vi "ADC INL_new - Copy.vi"(8 "error in (no error)":errorcluster, 9 "Sequence parameters":string[][](array[string])=[["Min limit", "Max limit", "Register sheet file", "Register Sheet"], ["", "", "CC2600.xls", "TX_BLE;Trim"], ["Reg write (addr;value)", "Operating frequency [Hz]", "", ""], ["NA", "2.44G", "", ""]], 10 "Run type":i32, 11 "Method parameters":T3={"Dev"={"Do not disturb DUT"=FALSE, "XOSC"=32000000.0, "Board type"="", "EM"="", "Configure tempboard"=TRUE, "Device specific info"=[], "Generic Object"=refnum}, "Method"={"Run type"=1, "Test name"="Current LPM2 4", "Comment"="", "Results folder"="", "AFC"=enum."Off", "Method name"="Current LPM2 4", "Method results"={"Excel brief report"=FALSE, "Spotfire report"=FALSE, "Starfish report"=FALSE}, "Operator"="", "Reference time"=timestamp(0 s since 1904-01-01), "AFC delay"=0.0, "Initialization"=enum."Enabled", "MD5 Sum"="", "HW addon board"=enum."None", "AFC Regsheet"="", "AFC Regfile"=path "", "dummy"=0.0}, "Inst"={"Instr"={"PS1"={"Name"="", "GPIB address"="", "VISA session"=""}, "PS2"={"Name"="", "GPIB address"="", "VISA session"=""}, "TC1"={"Name"="", "GPIB address"="", "VISA session"=""}, "TC2"={"Name"="", "GPIB address"="", "VISA session"=""}, "SA1"={"Name"="", "GPIB address"="", "VISA session"=""}, "SA2"={"Name"="", "GPIB address"="", "VISA session"=""}, "SG1"={"Name"="", "GPIB address"="", "VISA session"=""}, "SG2"={"Name"="", "GPIB address"="", "VISA session"=""}, "SG3"={"Name"="", "GPIB address"="", "VISA session"=""}, "MI1"={"Name"="", "GPIB address"="", "VISA session"=""}, "MI2"={"Name"="", "GPIB address"="", "VISA session"=""}, "SW SA"={"Name"="", "Controller addr"=""}, "SW SG"={"Name"="", "Controller addr"=""}, "MI3"={"Name"="", "GPIB address"="", "VISA session"=""}}, "Switchbox"={"RF Path"=0, "Cal compensation"=enum."TX", "Switchbox gain mode"="", "State"=enum."TX"}, "Instr to control (i.e. SA1)"="Default", "Intrument info string"=""}, "Sequence parameters"=[["Weight", "Min Limit", "Max Limit", "Register Sheet", "", "", "", "", "", "", "", "", ""], ["Vital", "", "1", "LPM2", "", "", "", "", "", "", "", "", ""], ["Resolution", "Reg write (addr;value)", "Chip mode", "Range", "", "", "", "", "", "", "", "", ""], ["u", "NA", "", "auto", "", "", "", "", "", "", "", "", ""]], "Cond"={"Temp logged"=25.0, "VDD1_PS1_6V"=-999.0, "VDD2_PS1_25V"=-999.0, "VDD4_PS2_25V"=-999.0, "VDD3_PS2_6V"=-999.0}, "Meas config"={"X-axis inner loop index"=32000000, "Y-axis outer loop index"=32000000, "X-axis"=[], "Y-axis"=[], "X-axis array req size"=32000000, "Y-axis array req size"=32000000, "Param description"=[], "Use meas clust for reporting"=FALSE, "Parameter index (page)"=0, "X-axis name"="", "Y-axis name"=""}} {"Cond"."VDD3_PS2_6V" format="%.3f"; "Cond"."VDD4_PS2_25V" format="%.3f"; "Cond"."VDD2_PS1_25V" format="%.3f"; "Cond"."VDD1_PS1_6V" format="%.3f"; "Method"."dummy" format="%.1p"; "Method"."AFC delay" format="%.1p"; "Dev"."XOSC" format="%.3p"}) -> (0 "error out":errorcluster, 1 "End method error":T2, 2 "Short Results":string[](array[string])=["0.00", "0.00", "0.00", "0.00"], 3 "Result summary":string[][](array[string])=[["Critical", "Output Power@2405 MHz", "-3", "4", "dBm"], ["Critical", "Output Power@2410 MHz", "-3", "4", "dBm"]])   [LabVIEW 2019]
doc: "[AutoDocStart]Performs crystal accuracy measurements. Measures the offset from ideal frequency. Primarily used for tuning XOSC capacitors and verifying XOSC trims.\n\nSweeping parameters: operating frequency, OSC override value and VDDR level\n\nResults: Offset frequency in ppm[AutoDocEnd]"
uses:
  User Lib/Utilities/Cluster definitions/Method input.ctl
  User Lib/Utilities/Cluster definitions/Device specific info.ctl
  User Lib/Utilities/Controls/Automatic Frequency Compensation types.ctl
  User Lib/Utilities/Controls/Method Reports.ctl
  User Lib/Utilities/Cluster definitions/Method Initialization.ctl
  User Lib/Utilities/Controls/HW addon boards.ctl
  User Lib/Utilities/Cluster definitions/Instr clust.ctl
  User Lib/Utilities/Switchbox control/SwitchBox_State._ENUMctl.ctl
  User Lib/Utilities/Cluster definitions/End method error cluster.ctl
  User Lib/Utilities/Cluster definitions/DUT vdd control.ctl
  User Lib/Utilities/Cluster definitions/DUT VDD4.ctl
  User Lib/Utilities/Cluster definitions/DUT VDD3.ctl
  User Lib/Utilities/Cluster definitions/DUT VDD2.ctl
  User Lib/Utilities/Cluster definitions/DUT VDD1.ctl
  User Lib/Generic chip methods/Classes/Generic_EM/Chameleon/Loki/Loki.lvclass
  <vilib>/Utility/error.llb/Clear Errors.vi
  User Lib/Generic chip methods/Classes/Generic_EM/Chameleon/65nm.lvclass
  C:/Kharon/User Lib/Generic chip methods/Classes/Generic_EM/Generic_EM/Generic_EM.lvclass
  User Lib/Generic chip methods/board_to_chip_type.vi
  User Lib/Generic chip methods/Classes/Get_Class_init.vi
  User Lib/Generic chip methods/Classes/Generic_EM/Generic_EM/Generic_EM.lvclass
panel:
  in  "Tab Control":T1(tab)
  out "output cluster":T11={"Average Hits \nper Code "=198.76479217603912, "Min DNL"=-0.30764433555407467, "Min INL"=-0.5231398172109945, "Max INL"=0.7801825995135989, "Max DNL"=0.8022935268616486, "DNL Range"=0.5549689312078616, "INL Range"=0.6516612083622967}
  out "ADC samples":u32[](array[numeric])
  out "Output Response [All DUTs]":u32[][](array[numeric])
  # "°C"
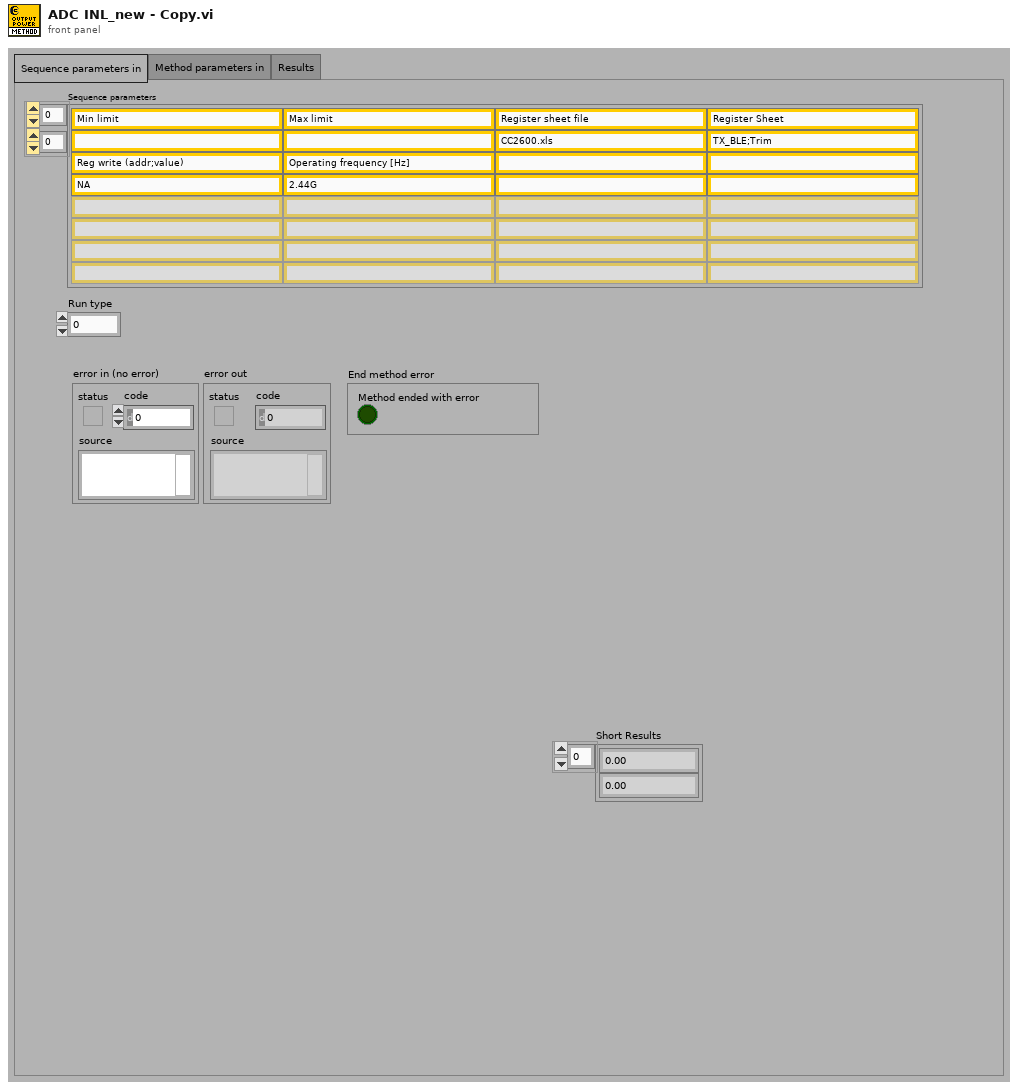
[diagram p1: front panel]
types:
  T1 = enum32{"Sequence parameters in", "Method parameters in", "Results"}
  T2 = typedef "End method error cluster.ctl" = cluster{"Method ended with error":bool}
  T3 = typedef "Method input.ctl" = cluster{"Dev":cluster{"Do not disturb DUT":bool, "XOSC":dbl, "Board type":string, "EM":string, "Configure tempboard":bool, "Device specific info":T4[], "Generic Object":refnum<class>}, "Method":cluster{"Run type":i32, "Test name":string, "Comment":string, "Results folder":string, "AFC":T5, "Method name":string, "Method results":T6, "Operator":string, "Reference time":timestamp, "AFC delay":dbl, "Initialization":T7, "MD5 Sum":string, "HW addon board":T8, "AFC Regsheet":string, "AFC Regfile":path, "dummy":dbl}, "Inst":T9, "Sequence parameters":string[][], "Cond":cluster{"Temp logged":dbl, "VDD1_PS1_6V":dbl, "VDD2_PS1_25V":dbl, "VDD4_PS2_25V":dbl, "VDD3_PS2_6V":dbl}, "Meas config":cluster{"X-axis inner loop index":i32, "Y-axis outer loop index":i32, "X-axis":string[], "Y-axis":string[], "X-axis array req size":i32, "Y-axis array req size":i32, "Param description":string[][], "Use meas clust for reporting":bool, "Parameter index (page)":i32, "X-axis name":string, "Y-axis name":string}}
  T4 = typedef "Device specific info.ctl" = cluster{"EM number":u8, "IP address":string, "Enabled":bool, "Slot no":u8, "RF path":u8, "EM name":string, "Wafer info":string, "AFC frequency ppm":dbl, "Register writes":string[][], "Meas data":string[][][], "Device comment":string}
  T5 = typedef "Automatic Frequency Compensation types.ctl" = enum16{"Off", "Compensate Instrument frequency", "Compensate DUT frequency", "Predictive - Compensate Instrument frequency", "Predictive - Compensate DUT frequency", "Do not skip re-init - Compensate Instrument frequency", "Do not skip re-init - Compensate DUT frequency"}
  T6 = typedef "Method Reports.ctl" = cluster{"Excel brief report":bool, "Spotfire report":bool, "Starfish report":bool}
  T7 = typedef "Method Initialization.ctl" = enum16{"Enabled", "Skip Instr and Device Init", "Enabled with Separate Flash", "Set PS, Device Init and Skip Instr Init", "Skip Device Init"}
  T8 = typedef "HW addon boards.ctl" = enum16{"None", "Current meas 5EM", "Stresstest 10EM"}
  T9 = typedef "Instr clust.ctl" = cluster{"Instr":cluster{"PS1":cluster{"Name":string, "GPIB address":string, "VISA session":refnum<visa-resource-name>}, "PS2":cluster{"Name":string, "GPIB address":string, "VISA session":refnum<visa-resource-name>}, "TC1":cluster{"Name":string, "GPIB address":string, "VISA session":refnum<visa-resource-name>}, "TC2":cluster{"Name":string, "GPIB address":string, "VISA session":refnum<visa-resource-name>}, "SA1":cluster{"Name":string, "GPIB address":string, "VISA session":refnum<visa-resource-name>}, "SA2":cluster{"Name":string, "GPIB address":string, "VISA session":refnum<visa-resource-name>}, "SG1":cluster{"Name":string, "GPIB address":string, "VISA session":refnum<visa-resource-name>}, "SG2":cluster{"Name":string, "GPIB address":string, "VISA session":refnum<visa-resource-name>}, "SG3":cluster{"Name":string, "GPIB address":string, "VISA session":refnum<visa-resource-name>}, "MI1":cluster{"Name":string, "GPIB address":string, "VISA session":refnum<visa-resource-name>}, "MI2":cluster{"Name":string, "GPIB address":string, "VISA session":refnum<visa-resource-name>}, "SW SA":cluster{"Name":string, "Controller addr":string}, "SW SG":cluster{"Name":string, "Controller addr":string}, "MI3":cluster{"Name":string, "GPIB address":string, "VISA session":refnum<visa-resource-name>}}, "Switchbox":cluster{"RF Path":i32, "Cal compensation":enum16{"TX", "RX", "Interferer", "No compensation", "Interferer2"}, "Switchbox gain mode":string, "State":T10}, "Instr to control (i.e. SA1)":string, "Intrument info string":string}
  T10 = typedef "SwitchBox_State._ENUMctl.ctl" = enum16{"TX", "RX", "SP:TX", "SP:RX", "SW:TX", "SW:RX"}
  T11 = cluster{"Average Hits \nper Code ":dbl, "Min DNL":dbl, "Min INL":dbl, "Max INL":dbl, "Max DNL":dbl, "DNL Range":dbl, "INL Range":dbl}
  T12 = cluster{"Path to Save plot":path, "Path to Raw Data plot":path}
  T13 = cluster{"Save INL/DNL Plot(Ramp)":bool, "Save SNR Plot":bool, "Save INL/DNL Plot(Sine)":bool, "Save INL/DNL Raw Data(Ramp)":bool, "Save SNR Raw Data":bool, "Save INL/DNL Raw Data(Sine)":bool, "Save DC Raw data":bool, "Save  Raw Data(Sine)":bool}
  T14 = typedef "DUT vdd control.ctl" = cluster{"VDD4 config":T15, "VDD3 config":T16, "VDD2 config":T17, "VDD1 config":T18}
  T15 = typedef "DUT VDD4.ctl" = u16
  T16 = typedef "DUT VDD3.ctl" = u16
  T17 = typedef "DUT VDD2.ctl" = u16
  T18 = typedef "DUT VDD1.ctl" = u16
  T19 = enum32{"NI Card Settings", "Memory Read Setting", "DC Capture", "ADC Ramp", "ADC Sine", "SNR", "Cap Calibration"}
  T20 = enum32{"Read from Memory", "Read .dat file", "NI Card Capture", "None"}
  T21 = typedef "TFW ResponseData.ctl" = cluster{"errorCode":u32, "executionTime":u32, "processedCmdWord":u32, "responsePar":u32[], "actionCode":u32, "cmdStatus":u16}
  T22 = cluster{"Min INL":dbl, "Max INL":dbl, "Min DNL":dbl, "Max DNL":dbl, "INL Range":dbl, "DNL Range":dbl, "Avg Hits/Code":dbl}
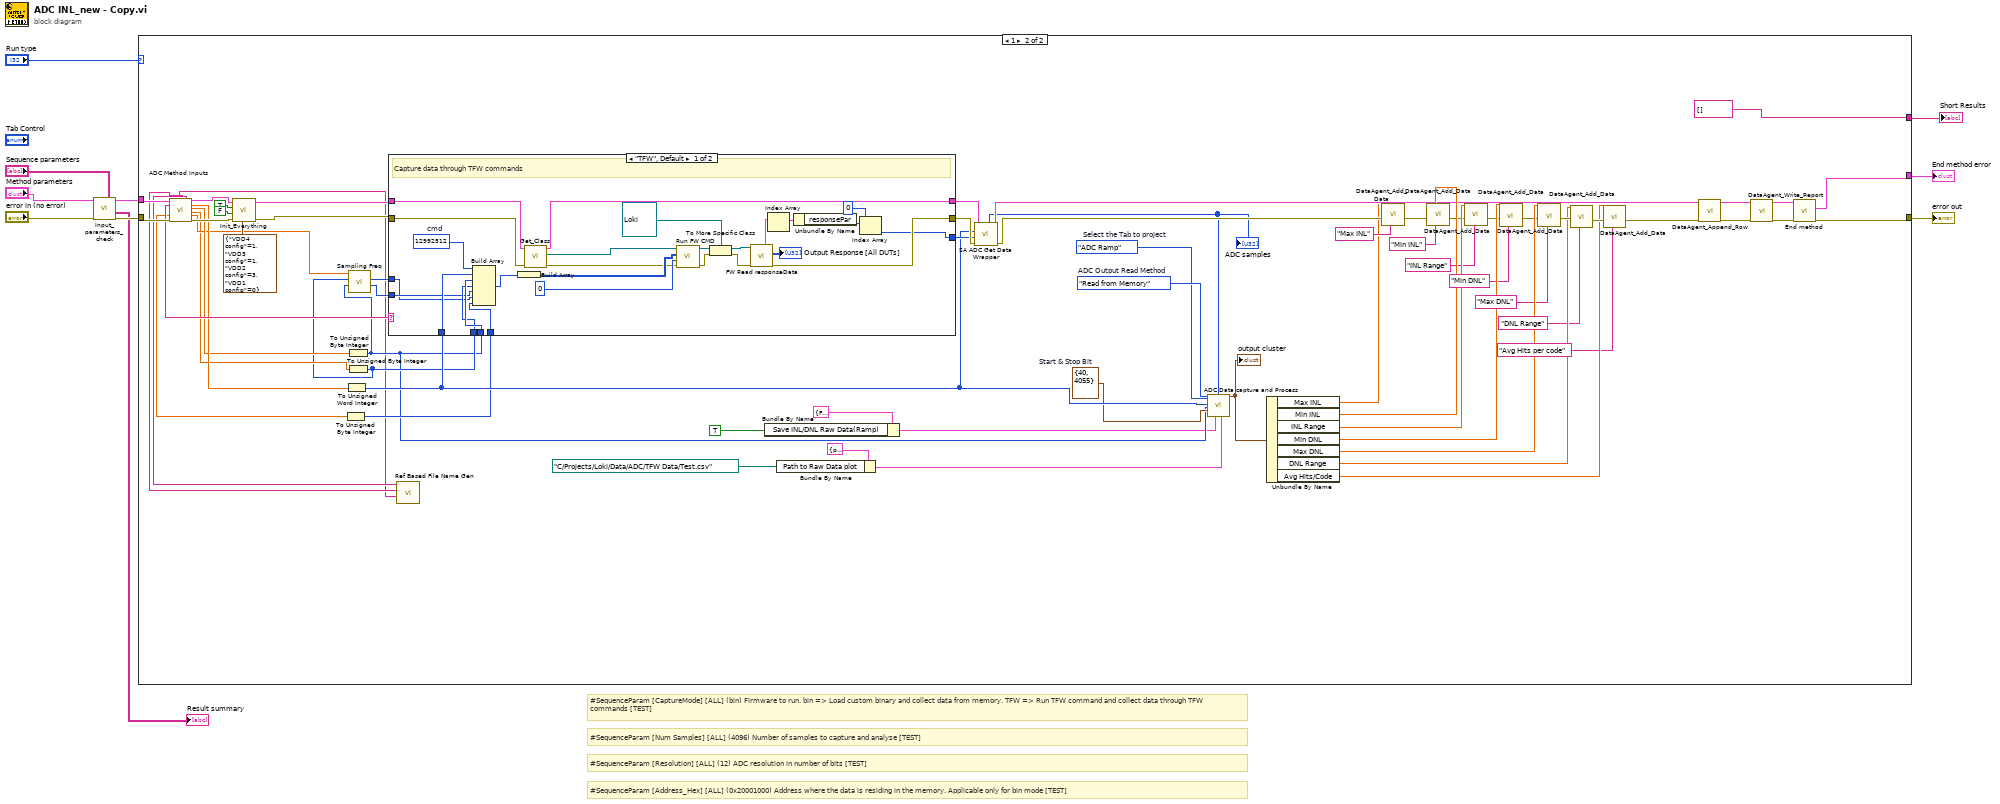
[diagram p0: block diagram]
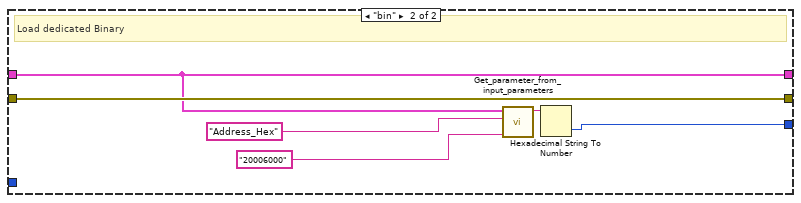
[diagram p3: hidden frame]
diagram:
  # "#SequenceParam [Num Samples] [ALL] (4096) Number of samples to capture and analyse [TEST]"
  # "#SequenceParam [CaptureMode] [ALL] (bin) Firmware to run. bin => Load custom binary and collect data from memory. TFW => Run TFW command and collect data through TFW commands [TEST]"
  # "#SequenceParam [Address_Hex] [ALL] (0x20001000) Address where the data is residing in the memory. Applicable only for bin mode [TEST]"
  # "#SequenceParam [Resolution] [ALL] (12) ADC resolution in number of bits [TEST]"
  n1 = call "Input_parameters_check.vi"("Sequence parameters"="Sequence parameters", "error in"="error in (no error)", "Method cluster in"="Method parameters") -> ("error out"=w9:errorcluster, "Result summary"=→"Result summary":string[][], "Method cluster out"=w5:T3)  [unwired: 6 in]
  n2 = case shown="1" "Run type" {
    tunnel: w9 -> [w11 w50]
    tunnel: [w11 w79] -> w10
    tunnel: w5 -> [_ w51]
    tunnel: [_ w78] -> w4
    tunnel: [_ string[] []] -> w1
    frame 0, Default {
      # "Run type 0 is only for formatting the result summary"
    }
    frame 1 {
      w52 = cluster{"Start":i32, "Stop":i32} {"Start"=40, "Stop"=4055}  # Start & Stop Bit
      w71 = T19."ADC Ramp"  # Select the Tab to project
      w72 = T20."Read from Memory"  # ADC Output Read Method
      n3 = call "ADC Method Inputs.vi"("Method cluster in"=w51, "error in (no error)"=w50) -> ("Capture Mode"=w47:string, "ADC Chnl No."=w38:dbl, "Sampling Freq String"=w34:string, "Resolution String"=w35:string, "Voltage Ref String"=w36:string, "Method cluster out"=w48:T3, "Num Samples"=w46:dbl, "Resolution"=w45:dbl, "Voltage Ref"=w43:dbl, "Sampling Freq"=w44:dbl, "error out"=w49:errorcluster)  [unwired: 2 in, 5 out]
      n4 = call "Init_Everything.vi"("VDD config"=T14 {"VDD4 config"=1, "VDD3 config"=1, "VDD2 config"=3, "VDD1 config"=0}, "error in"=w49, "Support current measurement?"=FALSE, "Override VDD Config"=TRUE, "Method cluster In"=w48) -> ("error out"=w74:errorcluster, "Method cluster out"=w73:T3)  [unwired: 3 in, 2 out]
      n5 = To Unsigned Byte Integer(number=w38) -> (unsigned 8bit integer=w39:u8)
      n6 = To Unsigned Word Integer(number=w46) -> (unsigned 16bit integer=w60:u16)
      n7 = To Unsigned Byte Integer(number=w45) -> (unsigned 8bit integer=w37:u8)
      n8 = To Unsigned Byte Integer(number=w43) -> (unsigned 8bit integer=w40:u8)
      n9 = call "Sampling Freq.vi"("Resolution"=w37, "Voltage Ref"=w40, "Sampling Freq"=w44) -> ("LGPT Count"=w42:u16, "SCOMP"=w41:u16)  [unwired: 7 in]
      n10 = case shown="\"TFW\", Default" w47 {
        tunnel: [w106 w107] -> w63
        tunnel: [w100 w112] -> w62
        tunnel: w74 -> [w99 w112]
        tunnel: w73 -> [w105 w107]
        tunnel: [w87 w108] -> w61
        tunnel: w60 -> [w86 _]
        tunnel: w37 -> [w85 _]
        tunnel: w40 -> [w84 _]
        tunnel: w42 -> [w83 _]
        tunnel: w41 -> [w82 _]
        tunnel: w39 -> [w81 _]
        frame "TFW", Default {
          w103 = u32 12992512  # cmd
          # "Capture data through TFW commands"
          n11 = Build Array(w103, w86, w85, w84, w83, w82, w81) -> (w102:u32[])
          n12 = Build Array(w102) -> (w101:u32[][])
          n13 = call "Get_Class.vi"("error in (no error)"=w99, "Method cluster in"=w105) -> ("error out"=w97:errorcluster, "Class Out"=w96:refnum<class "Generic_EM.lvclass">, "Method cluster out"=w106:T3)  [unwired: 6 in, 1 out]
          n14 = call-dynamic "Run FW CMD.vi"("error in (no error)"=w97, "Handler"=u8 0, "cmdBuf"=w101, "Generic_EM in"=w96) -> ("error out"=w92:errorcluster, "Generic_EM out"=w95:refnum<class "Generic_EM.lvclass">)  [unwired: 6 in]
          n15 = To More Specific Class(target class=refnum<class "Loki.lvclass"> refnum ("Loki in"), reference=w95, error in=w92) -> (specific class reference=w93:refnum<class "Loki.lvclass">, error out=w91:errorcluster)
          n16 = call "FW Read responseData.vi"("error in (no error)"=w91, "Loki in"=w93) -> ("error out"=w100:errorcluster, "Output Response [All DUTs]"=→"Output Response [All DUTs]":u32[][], "Response"=w89:T21[])  [unwired: 6 in, 1 out]
          n17 = Index Array(array=w89) -> (element=w90:T21)  [unwired: 1 in]
          n18 = Unbundle By Name(w90) -> ("responsePar"=w88:u32[])
          n19 = Index Array(array=w88, index=0) -> (element=w87:u32)
        }
        frame "bin" {
          # "Load dedicated Binary"
          n20 = call "Get_parameter_from_input_parameters.vi"("Default value (used if not specified on Front Panel)"="20006000", "Parameter name"="Address_Hex" ("SA_ param name"), "Method cluster (if input param empty)"=w107) -> ("value as String"=w111:string)  [unwired: 2 in, 6 out]
          n21 = Hexadecimal String To Number(string=w111) -> (number=w108:u32)  [unwired: 2 in, 1 out]
        }
      }
      n22 = call "Ref Based File Name Gen.vi"("Sampling Freq String"=w34, "Resolution String"=w35, "Voltage Ref String"=w36) -> ()  [unwired: 8 in, 1 out]
      n23 = Bundle By Name(cluster=T13 {"Save INL/DNL Plot(Ramp)"=FALSE, "Save SNR Plot"=FALSE, "Save INL/DNL Plot(Sine)"=FALSE, "Save INL/DNL Raw Data(Ramp)"=FALSE, "Save SNR Raw Data"=FALSE, "Save INL/DNL Raw Data(Sine)"=FALSE, "Save DC Raw data"=FALSE, "Save  Raw Data(Sine)"=FALSE} ("Save data"), "Save INL/DNL Raw Data(Ramp)"=TRUE ("Save SNR Plot")) -> (w15:T13)
      n24 = Bundle By Name(cluster=T12 {"Path to Save plot"=path "D:/Tenor_176P/DYN_PAR_C004/DAT/D001_TEMPP30C_VDD1.2_VDDA3.3_16B_SE_ADCA__vicA_aggX_PLT_CAP_200821_1740_33.jpg", "Path to Raw Data plot"=path "D:/Tenor_176P/DYN_PAR_C004/DAT/D001_TEMPP30C_VDD1.2_VDDA3.3_16B_SE_ADCA__vicA_aggX_RAW_DAT_200821_1740_33.csv"} ("path to save"), "Path to Raw Data plot"=path "C:/Projects/Loki/Data/ADC/TFW Data/Test.csv" ("Path to Save plot")) -> (w13:T12)
      n25 = call "SA ADC Get Data Wrapper.vi"("error in"=w62, "Data Address"=w61, "Num Samples"=w60, "Method cluster in"=w63) -> ("error out"=w66:errorcluster, "output cluster"=w65:T3, "ADC samples"=w64:u32[])  [unwired: 2 in, 3 out]
      "ADC samples" <- w64
      n26 = call "ADC Data capture and Process.vi"("ADC Output Read Method"=w72, "Select the Tab to project"=w71, "No.of samples"=w60, "Resolution"=w37, "Start & Stop Bit"=w52, "Save data"=w15, "Input Waveform"=w64, "path to save"=w13) -> ("Static Parameters (Ramp)"=w12:T22)  [unwired: 14 in, 5 out]
      "output cluster" <- w12
      n27 = Unbundle By Name(w12) -> ("Max INL"=w33:dbl, "Min INL"=w68:dbl, "INL Range"=w32:dbl, "Min DNL"=w31:dbl, "Max DNL"=w30:dbl, "DNL Range"=w24:dbl, "Avg Hits/Code"=w23:dbl)
      n28 = call "DataAgent_Add_Data.vi"("ColumnName"="Max INL" ("Default Value"), "Data"=w33, "error in (no error)"=w66) -> ("error out"=w56:errorcluster)  [unwired: 8 in]
      n29 = call "DataAgent_Add_Data.vi"("ColumnName"="Min INL" ("Default Value"), "Data"=w68, "error in (no error)"=w56) -> ("error out"=w29:errorcluster)  [unwired: 8 in]
      n30 = call "DataAgent_Add_Data.vi"("ColumnName"="INL Range", "Data"=w32, "error in (no error)"=w29) -> ("error out"=w28:errorcluster)  [unwired: 8 in]
      n31 = call "DataAgent_Add_Data.vi"("ColumnName"="Min DNL", "Data"=w31, "error in (no error)"=w28) -> ("error out"=w27:errorcluster)  [unwired: 8 in]
      n32 = call "DataAgent_Add_Data.vi"("ColumnName"="Max DNL", "Data"=w30, "error in (no error)"=w27) -> ("error out"=w26:errorcluster)  [unwired: 8 in]
      n33 = call "DataAgent_Add_Data.vi"("ColumnName"="DNL Range", "Data"=w24, "error in (no error)"=w26) -> ("error out"=w25:errorcluster)  [unwired: 8 in]
      n34 = call "DataAgent_Add_Data.vi"("ColumnName"="Avg Hits per code", "Data"=w23, "error in (no error)"=w25) -> ("error out"=w22:errorcluster)  [unwired: 8 in]
      n35 = call "DataAgent_Append_Row.vi"("error in (no error)"=w22, "Method cluster in"=w65) -> ("error out"=w58:errorcluster, "Method cluster out"=w59:T3)  [unwired: 8 in]
      n36 = call "DataAgent_Write_Report.vi"("error in (no error)"=w58, "Method cluster in"=w59) -> ("error out"=w76:errorcluster, "Method cluster out"=w75:T3)  [unwired: 8 in]
      n37 = call "End method.vi"("error in"=w76, "Method cluster in"=w75) -> ("error out"=w79:errorcluster, "End method error"=w78:T2)  [unwired: 7 in, 1 out]
    }
  }
  "error out" <- w10
  "End method error" <- w4
  "Short Results" <- w1
